vi "LatLongUpperLowerBounds.vi"(0 "Latitude":dbl, 1 "Longitude":dbl) -> (2 "Lat Upper":dbl, 3 "Lat Lower":dbl, 4 "Long Upper":dbl, 5 "Long Lower":dbl)   [LabVIEW 2015]
doc: "Creates upper and lower bounds for the latitude and longitude values. If the current location is within range of these bounds then the waypoint has been reached and the next waypoint is taken. If not then the waypoint remains the same."
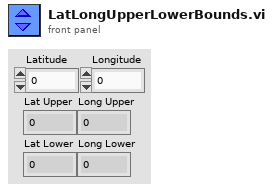
[diagram p1: front panel]
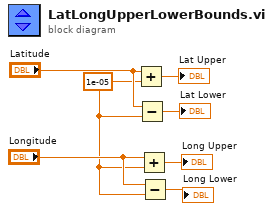
[diagram p0: block diagram]
diagram:
  w5 = 1e-05 ("y")
  n1 = Add(x="Latitude", y=w5) -> (x+y=→"Lat Upper":dbl)
  n2 = Subtract(x="Latitude", y=w5) -> (x-y=→"Lat Lower":dbl)
  n3 = Add(x="Longitude", y=w5) -> (x+y=→"Long Upper":dbl)
  n4 = Subtract(x="Longitude", y=w5) -> (x-y=→"Long Lower":dbl)
